vi "ThreadCfg - Allow Period Config.vi"(7 "rxPacket?":bool, 10 "threadPeriodRef":T2=enum."Async") -> (1 "pclDecimationState":T1(ring), 2 "loopPeriodState":T1(ring))   [LabVIEW 2016, in "UDP-Custom-Device System Explorer.lvlib"]
uses:
  UDP-Custom-Device System Explorer.lvlib
  Types/Threading/Thread Sync Reference.ctl
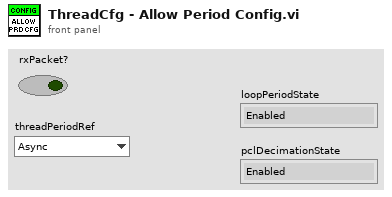
[diagram p1: front panel]
types:
  T1 = enum8{"Enabled", "Disabled", "Disabled and Grayed Out"}
  T2 = typedef "UDP-Custom-Device System Explorer.lvlib/Thread Sync Reference.ctl" = enum16{"PCL", "Async"}
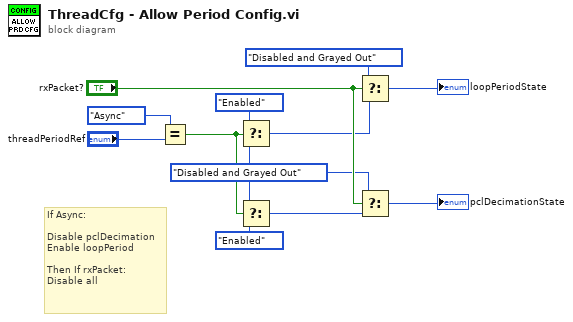
[diagram p0: block diagram]
diagram:
  w1 = T1."Disabled and Grayed Out" ("Disabled")
  # "If Async:\n\nDisable pclDecimation\nEnable loopPeriod\n\nThen If rxPacket:\nDisable all"
  n1 = Equal?(x=Thread_Sync_Reference."Async", y="threadPeriodRef") -> (x = y?=w4:bool)
  n2 = Select(t=T1."Enabled" ("Disabled"), s=w4, f=w1) -> (s? t:f=w2:T1)
  n3 = Select(t=w1, s=w4, f=T1."Enabled" ("Disabled")) -> (s? t:f=w3:T1)
  n4 = Select(t=T1."Disabled and Grayed Out" ("Disabled"), s="rxPacket?", f=w2) -> (s? t:f=→"loopPeriodState":T1)
  n5 = Select(t=w1, s="rxPacket?", f=w3) -> (s? t:f=→"pclDecimationState":T1)
